vi "Write Profile.vi"(8 "error in (no error)":errorcluster, 10 "profile":enum16{"Linear", "Half cosine"}(ring), 11 "SV Signal in":refnum<class "SV Signal.lvclass">) -> (0 "error out":errorcluster, 3 "SV Signal out":refnum<class "SV Signal.lvclass">)   [LabVIEW 2017, in "SV Signal.lvclass"]
uses:
  <vilib>/addons/_NISVFA/_Generation/Signal Generation/SV Signal/SV Signal.lvclass
  <vilib>/addons/_NISVFA/_Generation/Signal Generation/SV Signal/SV Signal.lvclass/SV Signal.ctl
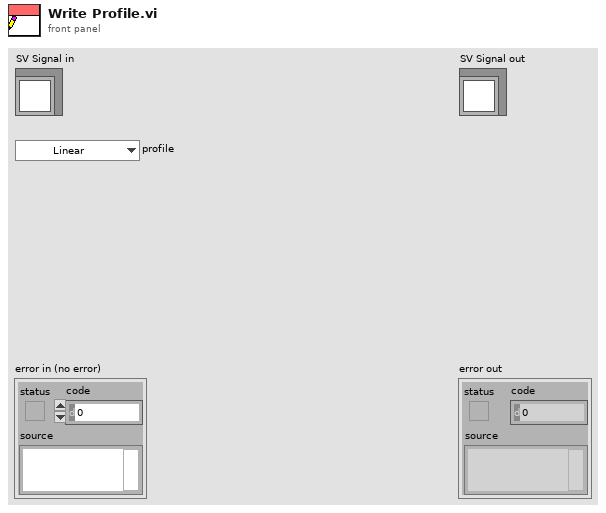
[diagram p1: front panel]
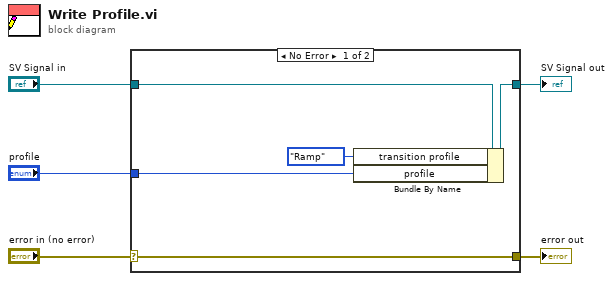
[diagram p0: block diagram]
diagram:
  n1 = case shown="No Error" "error in (no error)" {
    selector: "error in (no error)" -> [w10 w11]
    tunnel: [w10 w11] -> w4
    tunnel: [w8 w12] -> w2
    tunnel: "SV Signal in" -> [w9 w12]
    tunnel: "profile" -> [w7 _]
    frame No Error {
      n2 = Bundle By Name(cluster=w9, "transition profile"=enum16{"Immediate", "Next optimum", "Ramp"}."Ramp", "profile"=w7) -> (w8:refnum<class "SV Signal.lvclass">)
    }
    frame Error {
    }
  }
  "error out" <- w4
  "SV Signal out" <- w2
